vi "isUnregistered.vi"(8 "error in (no error)":errorcluster, 10 "name":string, 11 "Event in":refnum<class "Event.lvclass">) -> (0 "error out":errorcluster, 2 "unregistered":bool, 3 "Event out":refnum<class "Event.lvclass">)   [LabVIEW 2011, in "Events.lvlib" / "Event.lvclass"]
uses:
  Event.lvclass
  Event.lvclass/Event.ctl
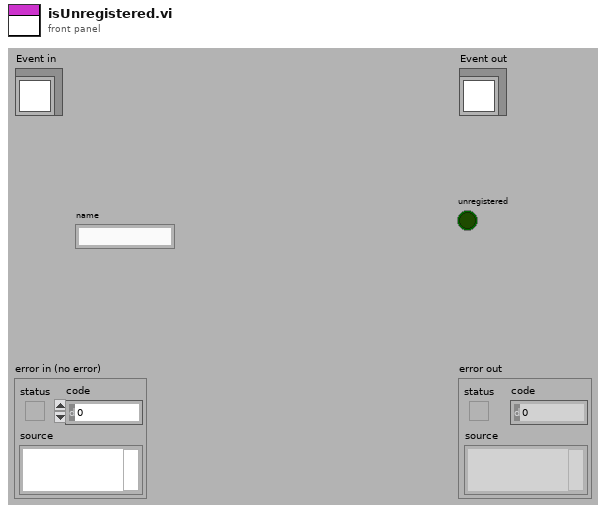
[diagram p1: front panel]
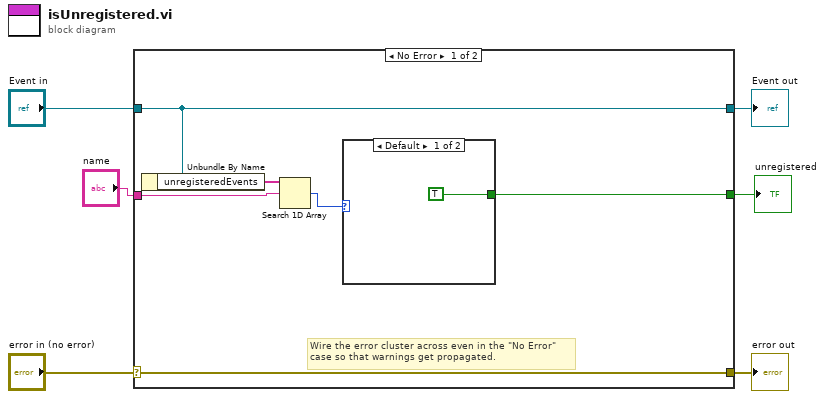
[diagram p0: block diagram]
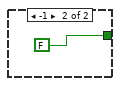
[diagram p2: hidden frame]
diagram:
  n1 = case shown="No Error" "error in (no error)" {
    selector: "error in (no error)" -> [w12 w16]
    tunnel: [w12 w16] -> w5
    tunnel: [w11 w15] -> w3
    tunnel: "Event in" -> [w11 w15]
    tunnel: "name" -> [w9 _]
    tunnel: [w7 _] -> w1
    frame No Error {
      # "Wire the error cluster across even in the \"No Error\"\ncase so that warnings get propagated."
      n2 = Unbundle By Name(w11) -> ("unregisteredEvents"=w10:string[])
      n3 = Search 1D Array(1D array=w10, element=w9) -> (index of element=w8:i32)  [unwired: 1 in]
      n4 = case shown="Default" w8 {
        tunnel: [TRUE FALSE] -> w7
        frame Default {
        }
        frame -1 {
        }
      }
    }
    frame Error {
    }
  }
  "error out" <- w5
  "Event out" <- w3
  "unregistered" <- w1
